vi "DpcWaitForTransaction.vi"(8 "Error In":errorcluster, 10 "Task ID":u16, 11 "Device Handle":u32) -> (0 "Error Out":errorcluster, 3 "Device Handle":u32)   [LabVIEW 2011, in "LVH-Adept.lvlib" / "DPCUTIL.lvlib"]
doc: "DPCAPI BOOL DpcOpenData(HANDLE * phif, char * szdvc, ERC * perc, TRID * ptrid);"
uses:
  DPCUTIL.lvlib
  Private/Type Defs/Error.ctl
  Resources/dpcutil.dll
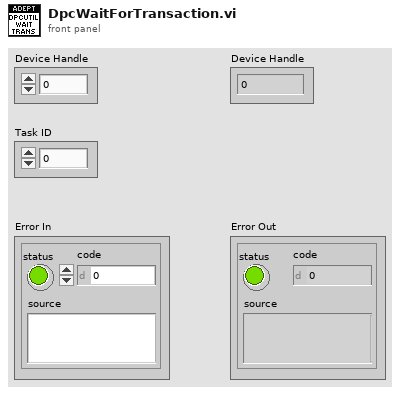
[diagram p1: front panel]
types:
  T1 = typedef "LVH-Adept.lvlib/DPCUTIL.lvlib/Error.ctl" = enum16{"Unknown", "Open Data", "Wait For Transaction", "Put Reg", "Get Reg", "Close Data"}
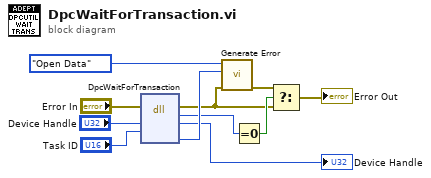
[diagram p0: block diagram]
diagram:
  n1 = dll-call lib="C:/github/labviewhacker/LVH-Adept/LabVIEW/vi.lib/LabVIEW Hacker/Adept/Private/Resources/dpcutil.*" fn="DpcWaitForTransaction"(error in="Error In", "hif"="Device Handle", "trid"="Task ID") -> (error out=w1:errorcluster, "return type"=w5:i32, "hif"=→"Device Handle":u32, "perc"=w6:i32)  [unwired: 4 in, 1 out]
  n2 = call "Generate Error.vi"("Error In"=w1, "Adept Error Code"=w6, "DPCUTIL Error"=Error."Open Data") -> ("Error Out"=w9:errorcluster)  [unwired: 8 in]
  n3 = Equal To 0?(x=w5) -> (x = 0?=w11:bool)
  n4 = Select(t=w9, s=w11, f=w1) -> (s? t:f=→"Error Out":errorcluster)
